vi "Start 1Hz livestream video from CamServer (TCP CLIENT).vi"(1 "Quality":i32=750 min=0 max=1000, 2 "Camera":T2="Travcam", 3 "Video name":string, 4 "Video directory path":path, 5 "Write video":bool, 6 "TCP/IP port":u16=80) -> (0 "Error out":errorcluster)   [LabVIEW 2015]
doc: "Starts a video livestream from the camera server. The stream can also be saved to a local directory."
uses:
  Camera enum/Camera enum.ctl
  <vilib>/vision/Avi.llb/IMAQ AVI2 Refnum.ctl
  Globals/CamServer global.vi
panel:
  in  "Stop":bool
  out "Video":T1(plugin-control)
  # "PN 01/09/15"
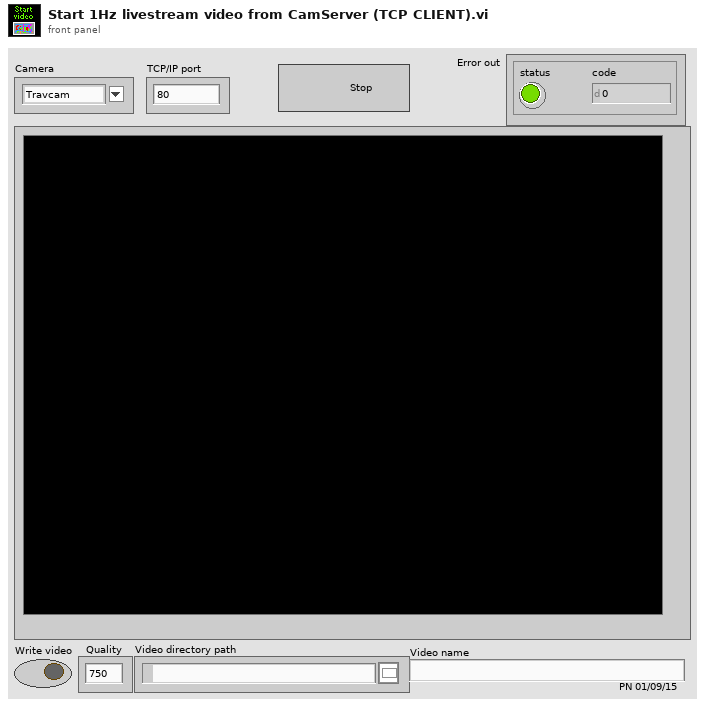
[diagram p1: front panel]
types:
  T1 = typedef "IMAQ Image.ctl" = refnum<image>
  T2 = typedef "Camera enum.ctl" = string
  T3 = typedef "IMAQ AVI2 Refnum.ctl" = refnum<k20>
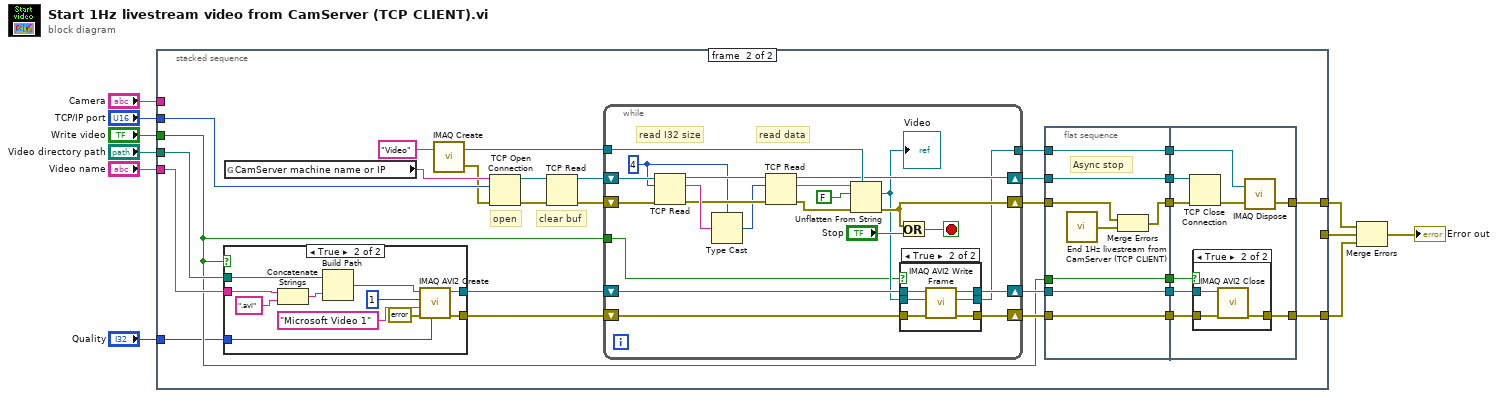
[diagram p0: block diagram]
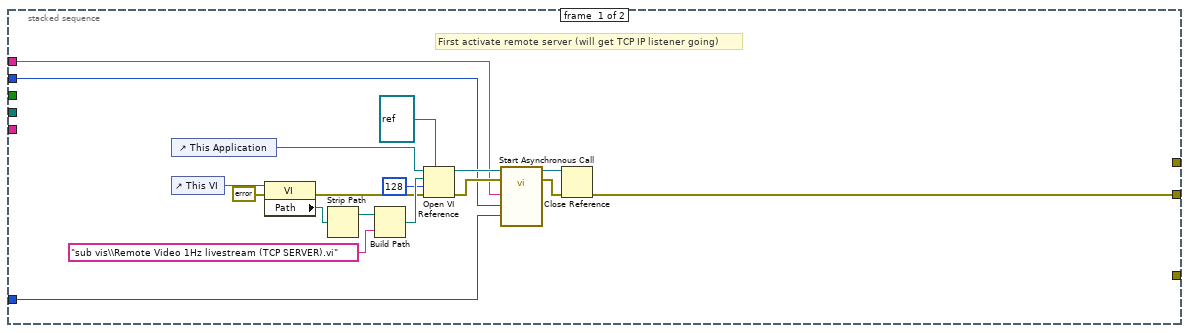
[diagram p2: hidden frame]
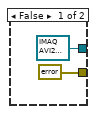
[diagram p3: hidden frame]
diagram:
  n1 = stacked-sequence {
    tunnel: "Camera" -> [w14 _]
    tunnel: "TCP/IP port" -> [w13 w56]
    tunnel: "Write video" -> [_ w31]
    tunnel: [w12 _] -> w7
    tunnel: [_ w41] -> w6
    tunnel: [_ w34] -> w4
    tunnel: "Video name" -> [_ w33]
    tunnel: "Video directory path" -> [_ w32]
    tunnel: "Quality" -> [w11 w29]
    frame #0 {
      # "First activate remote server (will get TCP IP listener going)"
      n2 = control-ref of="This Application"() -> (w23:refnum<vi>)
      n3 = control-ref of="This VI"() -> (w28:refnum<vi>)
      n4 = property class="VI"(reference=w28, error in=errorcluster {"status"=FALSE, "code"=0, "source"=""} ("error in (no error)")) -> (error out=w25:errorcluster, "Path"=w21:path)  [unwired: 1 out]
      n5 = Strip Path(path=w21) -> (stripped path=w20:path)  [unwired: 1 out]
      n6 = Build Path(base path=w20, name or relative path="sub vis\\Remote Video 1Hz livestream (TCP SERVER).vi") -> (appended path=w26:path)
      n7 = Open VI Reference(type specifier VI Refnum (for type only)=refnum<vi> refnum, application reference (local)=w23, vi path=w26, options=128, error in (no error)=w25) -> (vi reference=w19:refnum<vi>, error out=w18:errorcluster)  [unwired: 1 in]
      n8 = call-by-ref "Start Asynchronous Call"(reference=w19, error in=w18, "Quality"=w11, "TCP/IP port"=w13, "Camera"=w14) -> (reference out=w16:refnum<vi>, error out=w15:errorcluster)  [unwired: 1 out]
      n9 = Close Reference(reference=w16, error in (no error)=w15) -> (error out=w12:errorcluster)
    }
    frame #1 {
      # "open"
      # "clear buf"
      n10 = case shown="True" w31 {
        tunnel: [T3 refnum ("AVI Refnum") w69] -> w40
        tunnel: [errorcluster {"status"=FALSE, "code"=0, "source"=""} ("error out") w68] -> w39
        tunnel: w33 -> [_ w61]
        tunnel: w32 -> [_ w60]
        tunnel: w29 -> [_ w59]
        frame False {
        }
        frame True {
          n11 = Concatenate Strings(w61, ".avi" ("name or relative path")) -> (w63:string)
          n12 = Build Path(base path=w60, name or relative path=w63) -> (appended path=w62:path)
          n13 = call "IMAQ AVI2 Create"("Quality"=w59, "error in (no error)"=errorcluster {"status"=FALSE, "code"=0, "source"=""} ("error in"), "Codec"="Microsoft Video 1", "Frames Per Second"=u32 1, "AVI Path"=w62) -> ("error out"=w68:errorcluster, "AVI Refnum"=w69:T3)  [unwired: 5 in]
        }
      }
      n14 = global read "CamServer global.vi" "CamServer machine name or IP"() -> (w55:string)
      n15 = call "IMAQ Create"("Image Name"="Video") -> ("New Image"=w49:T1, "error out"=w48:errorcluster)  [unwired: 4 in]
      n16 = TCP Open Connection(address=w55, remote port or service name=w56, error in (no error)=w48) -> (connection ID=w53:refnum<k5>, error out=w54:errorcluster)  [unwired: 2 in]
      n17 = TCP Read(connection ID=w53, error in (no error)=w54) -> (connection ID out=w51:refnum<k5>, error out=w52:errorcluster)  [unwired: 3 in, 1 out]
      n18 = while {
        shift-right: [w101] -> w47
        shift-left: w51 -> [w112]
        shift-right: [w100] -> w46
        shift-left: w52 -> [w110]
        tunnel: w49 -> [w103]
        tunnel: [w91] -> w45
        shift-right: [w95] -> w35
        shift-left: w39 -> [w94]
        shift-right: [w96] -> w38
        shift-left: w40 -> [w97]
        tunnel: w31 -> [w92]
        stop <- w98 stop-if-true
        w102 = 4
        # "read data"
        # "read I32 size"
        n19 = TCP Read(connection ID=w112, bytes to read=w102, error in (no error)=w110) -> (connection ID out=w109:refnum<k5>, data out=w111:string, error out=w108:errorcluster)  [unwired: 2 in]
        n20 = Type Cast(type=w102, x=w111) -> (*(type *) &x=w107:i32)
        n21 = TCP Read(connection ID=w109, bytes to read=w107, error in (no error)=w108) -> (connection ID out=w101:refnum<k5>, data out=w106:string, error out=w104:errorcluster)  [unwired: 2 in]
        n22 = Unflatten From String(type=w103, binary string=w106, data includes array or string size? (T)=FALSE, error in (no error)=w104) -> (value=w93:T1, error out=w100:errorcluster)  [unwired: 1 in, 1 out]
        "Video" <- w93
        n23 = Or(x=w100, y="Stop") -> (x .or. y?=w98:bool)
        n24 = case shown="True" w92 {
          tunnel: w97 -> [w115 w121]
          tunnel: w93 -> [w113 w120]
          tunnel: [w115 w119] -> w96
          tunnel: [w114 w118] -> w95
          tunnel: w94 -> [w114 w117]
          tunnel: [w113 w116] -> w91
          frame False {
          }
          frame True {
            n25 = call "IMAQ AVI2 Write Frame"("error in (no error)"=w117, "Image"=w120, "AVI Refnum"=w121) -> ("error out"=w118:errorcluster, "Image Out (duplicate)"=w116:T1, "AVI Refnum (duplicate)"=w119:T3)  [unwired: 6 in]
          }
        }
      }
      n26 = flat-sequence {
        tunnel: w45 -> [w76]
        tunnel: w46 -> [w74]
        tunnel: w47 -> [w77]
        tunnel: [w77] -> w44
        tunnel: [w73] -> w43
        tunnel: [w76] -> w42
        tunnel: w38 -> [w72]
        tunnel: [w72] -> w37
        tunnel: w35 -> [w71]
        tunnel: [w71] -> w36
        tunnel: w31 -> [w70]
        tunnel: [w70] -> w30
        tunnel: w44 -> [w86]
        tunnel: w43 -> [w85]
        tunnel: w42 -> [w83]
        tunnel: [w82] -> w41
        tunnel: w37 -> [w81]
        tunnel: w36 -> [w80]
        tunnel: [w79] -> w34
        tunnel: w30 -> [w78]
        frame #0 {
          # "Async stop"
          n27 = call "End 1Hz livestream from CamServer (TCP CLIENT).vi"() -> ("Error out"=w75:errorcluster)  [unwired: 1 in]
          n28 = Merge Errors(w74, w75) -> (w73:errorcluster)
        }
        frame #1 {
          n29 = TCP Close Connection(connection ID=w86, error in (no error)=w85) -> (error out=w84:errorcluster)  [unwired: 1 in, 1 out]
          n30 = case shown="True" w78 {
            tunnel: w80 -> [w87 w90]
            tunnel: [w87 w89] -> w79
            tunnel: w81 -> [_ w88]
            frame False {
            }
            frame True {
              n31 = call "IMAQ AVI2 Close"("error in (no error)"=w90, "AVI Refnum"=w88) -> ("error out"=w89:errorcluster)  [unwired: 9 in]
            }
          }
          n32 = call "IMAQ Dispose"("Image"=w83, "error in (no error)"=w84) -> ("error out"=w82:errorcluster)  [unwired: 4 in]
        }
      }
    }
  }
  n33 = Merge Errors(w6, w7, w4) -> (→"Error out":errorcluster)
